vi "总磷测量数据储存.vi"   [LabVIEW 2016, in "斯坦道总磷.lvlib"]
types:
  T1 = cluster{"时间标识":timestamp, "监测值":sgl, "单位":u16, "数据标识":string, "因子编码":u32, "标样参考值":sgl, "F0":sgl, "F1":sgl, "F2":sgl, "F3":sgl, "F4":sgl, "F5":sgl, "F6":sgl, "F7":sgl, "X":sgl, "温度":sgl, "湿度":sgl, "量程标识":string}
  T2 = enum16{"维护数据", "水样测试", "标样核查", "零点核查", "跨度核查", "空白测试", "平行样测试", "加标回收", "空白校准", "标样校准", "初始化（清洗）"}
  T3 = cluster{"运行模式":enum16{"维护模式", "常规模式", "应急模式", "质控模式"}, "质控频次":enum16{"关闭", "每天", "星期一", "星期二", "星期三", "星期四", "星期五", "星期六", "星期日"}, "空白核查时间":u16, "跨度核查时间":u16, "24H周期设置":bool[]}
  T4 = cluster{"系统时间":timestamp, "工作状态":enum16{"空闲", "水样测试", "标样核查", "零点核查", "跨度核查", "空白测试", "平行样测试", "加标回收", "空白校准", "标样校准", "初始化（清洗）"}, "测量模式":enum16{"待机", "连续模式", "周期模式", "定点模式", "受控模式", "手动模式"}, "告警代码":enum16{"无告警", "缺试剂告警", "缺水样告警", "缺蒸馏水告警", "缺标液告警", "仪表漏液告警", "标定异常告警", "超量程告警", "加热异常", "低试剂预警", "超上限告警", "超下限告警", "仪表内部其他异常", "滴定异常告警", "电极异常告警", "量程切换告警", "参数设置告警", "PH电极电位异常", "电导率电极异常", "浊度光度异常", "溶解氧电极异常", "溶解氧光强异常", "温度异常告警", "PH异常告警", "溶解氧异常告警", "电导率异常告警", "浊度异常告警", "叶绿素异常告警", "藻密度异常告警", "蓝绿藻异常告警", "ORP异常告警", "氨氮异常告警", "清洁刷异常告警", "SD卡异常告警", "蓝牙异常告警", "Wifi异常告警", "流程异常告警"}, "故障代码":enum16{"无故障", "电机故障", "温度故障", "通讯故障", "滴定故障"}, "日志代码":u16, "软件版本":u16, "F0":sgl, "F1":sgl, "F2":sgl, "F3":sgl, "T":sgl, "H":sgl, "id":u16, "flowid":u16, "量程":u16, "总磷控温温度1":sgl, "营养盐控温温度2":sgl, "ADC":sgl}
  T5 = enum16{"空闲", "水样测试", "标样核查", "零点核查", "跨度核查", "空白测试", "平行样测试", "加标回收", "空白校准", "标样校准", "初始化（清洗）"}
  T6 = cluster{"因子编码":u32, "单位":u16, "标样参考值":sgl, "水样数据时间":timestamp, "水样实测值":sgl, "水样数据标识":string, "标样数据时间":timestamp, "标样实测值":sgl, "标样数据标识":string, "空白数据时间":timestamp, "空白实测值":sgl, "空白数据标识":string, "零点核查数据时间":timestamp, "零点核查实测值":sgl, "零点核查数据标识":string, "跨度核查数据时间":timestamp, "跨度核查实测值":sgl, "跨度核查数据标识":string, "加标回收数据时间":timestamp, "加标回收实测值":sgl, "加标回收数据标识":string, "平行样数据时间":timestamp, "平行样实测值":sgl, "平行样数据标识":string, "F0":sgl, "F1":sgl, "F2":sgl, "F3":sgl, "F4":sgl, "F5":sgl, "F6":sgl, "F7":sgl, "温度":sgl, "湿度":sgl, "X值":sgl}
  T7 = cluster{"总磷跨度值":dbl, "总磷零点标准液浓度":dbl, "总磷跨度标准液浓度":dbl, "总磷标准液标准浓度":dbl}
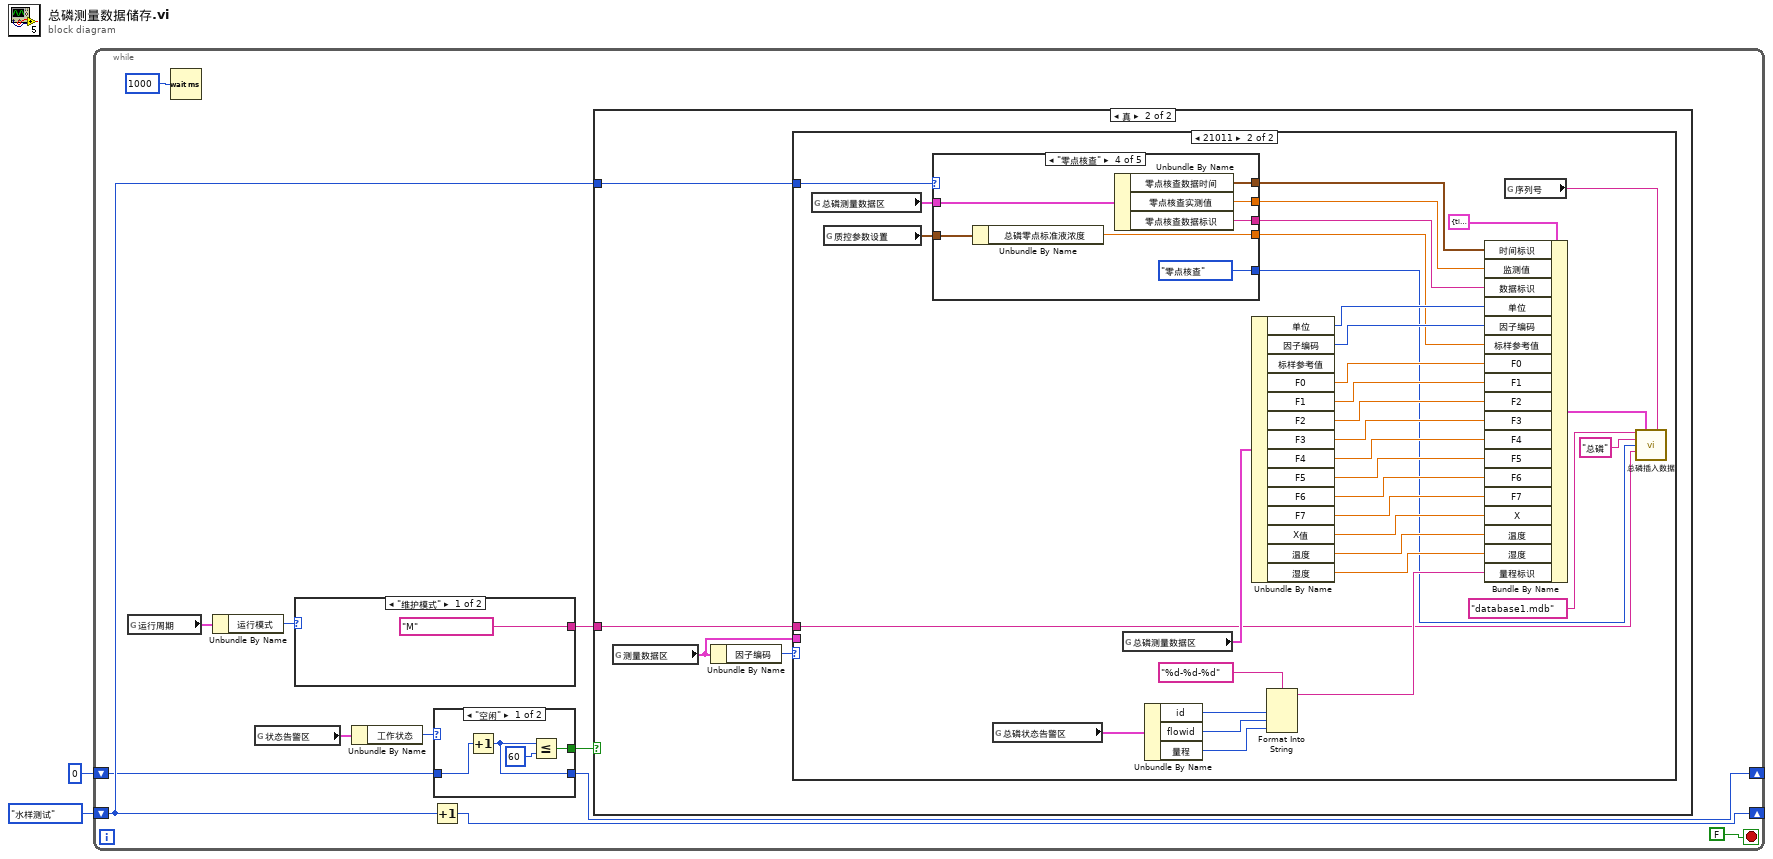
[diagram p0: block diagram]
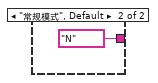
[diagram p3: hidden frame]
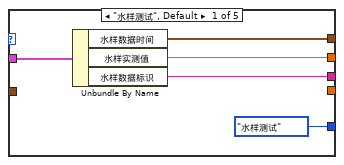
[diagram p6: hidden frame]
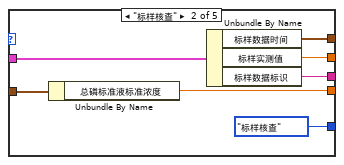
[diagram p7: hidden frame]
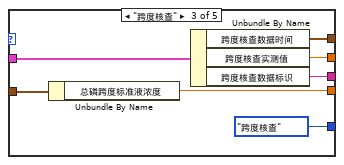
[diagram p8: hidden frame]
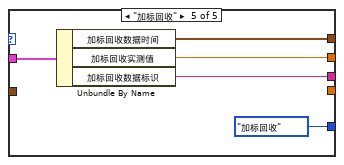
[diagram p9: hidden frame]
diagram:
  n1 = while {
    shift-right: [w12] -> _
    shift-left: enum16{"水样测试", "标样核查", "跨度核查", "零点核查", "加标回收"}."水样测试" ("测量模式") -> [w11]
    shift-right: [w5] -> _
    shift-left: u32 0 ("等待时间（毫秒）") -> [w6]
    stop <- FALSE stop-if-true
    n2 = global read "总磷断电保存全局变量.vi" "运行周期"() -> (w10:T3)
    n3 = Wait (ms)(milliseconds to wait=u32 1000 ("等待时间（毫秒）")) -> ()  [unwired: 1 out]
    n4 = Unbundle By Name(w10) -> ("运行模式"=w9:enum16{"维护模式", "常规模式", "应急模式", "质控模式"})
    n5 = global read "VAR总磷全局变量.vi" "状态告警区"() -> (w8:T4)
    n6 = case shown="\"维护模式\"" w9 {
      tunnel: ["M" ("数据标记表") "N" ("数据标记表")] -> w13
      frame "维护模式" {
      }
      frame "常规模式", Default {
      }
    }
    n7 = Unbundle By Name(w8) -> ("工作状态"=w7:T5)
    n8 = Increment(x=w11) -> (x+1=w12:enum16{"水样测试", "标样核查", "跨度核查", "零点核查", "加标回收"})
    n9 = case shown="\"空闲\"" w7 {
      tunnel: w6 -> [w18 _]
      tunnel: [w17 _] -> w5
      tunnel: [w15 _] -> w4
      frame "空闲" {
        n10 = Increment(x=w18) -> (x+1=w17:u32)
        n11 = Less Or Equal?(x=w17, y=u32 60) -> (x <= y?=w15:bool)
      }
      frame "水样测试", Default {
      }
    }
    n12 = case shown="真" w4 {
      tunnel: w13 -> [_ w22]
      tunnel: w11 -> [_ w21]
      frame False {
      }
      frame True {
        n13 = global read "VAR总磷全局变量.vi" "测量数据区"() -> (w24:T6)
        n14 = Unbundle By Name(w24) -> ("因子编码"=w23:u32)
        n15 = case shown="21011" w23 {
          tunnel: w24 -> [_ _]
          tunnel: w22 -> [_ w29]
          tunnel: w21 -> [_ w28]
          frame Default {
          }
          frame 21011 {
            n16 = global read "VAR总磷全局变量.vi" "总磷测量数据区"() -> (w57:T6)
            n17 = global read "总磷断电保存全局变量.vi" "质控参数设置"() -> (w26:T7)
            n18 = case shown="\"零点核查\"" w28 {
              tunnel: w57 -> [w63 w70 w77 w84 w89]
              tunnel: [w62 w69 w76 w83 w88] -> w33
              tunnel: [w61 w68 w75 w82 w87] -> w34
              tunnel: [w60 w67 w74 w81 w86] -> w35
              tunnel: [T2."水样测试" ("测量模式") T2."标样核查" ("测量模式") T2."跨度核查" ("测量模式") T2."零点核查" ("测量模式") T2."加标回收" ("测量模式")] -> w32
              tunnel: w26 -> [_ w65 w72 w79 _]
              tunnel: [_ w64 w71 w78 _] -> w25
              frame "水样测试", Default {
                n19 = Unbundle By Name(w63) -> ("水样数据时间"=w62:timestamp, "水样实测值"=w61:sgl, "水样数据标识"=w60:string)
              }
              frame "标样核查" {
                n20 = Unbundle By Name(w65) -> ("总磷标准液标准浓度"=w64:dbl)
                n21 = Unbundle By Name(w70) -> ("标样数据时间"=w69:timestamp, "标样实测值"=w68:sgl, "标样数据标识"=w67:string)
              }
              frame "跨度核查" {
                n22 = Unbundle By Name(w72) -> ("总磷跨度标准液浓度"=w71:dbl)
                n23 = Unbundle By Name(w77) -> ("跨度核查数据时间"=w76:timestamp, "跨度核查实测值"=w75:sgl, "跨度核查数据标识"=w74:string)
              }
              frame "零点核查" {
                n24 = Unbundle By Name(w79) -> ("总磷零点标准液浓度"=w78:dbl)
                n25 = Unbundle By Name(w84) -> ("零点核查数据时间"=w83:timestamp, "零点核查实测值"=w82:sgl, "零点核查数据标识"=w81:string)
              }
              frame "加标回收" {
                n26 = Unbundle By Name(w89) -> ("加标回收数据时间"=w88:timestamp, "加标回收实测值"=w87:sgl, "加标回收数据标识"=w86:string)
              }
            }
            n27 = global read "VAR总磷全局变量.vi" "总磷状态告警区"() -> (w27:T4)
            n28 = global read "VAR总磷全局变量.vi" "总磷测量数据区"() -> (w40:T6)
            n29 = Unbundle By Name(w27) -> ("id"=w58:u16, "flowid"=w42:u16, "量程"=w41:u16)
            n30 = Unbundle By Name(w40) -> ("单位"=w56:u16, "因子编码"=w55:u32, "F0"=w54:sgl, "F1"=w53:sgl, "F2"=w52:sgl, "F3"=w51:sgl, "F4"=w50:sgl, "F5"=w49:sgl, "F6"=w48:sgl, "F7"=w47:sgl, "X值"=w46:sgl, "温度"=w45:sgl, "湿度"=w44:sgl)  [unwired: 1 out]
            n31 = Format Into String(format string="%d-%d-%d" ("格式字符串"), w58, w42, w41) -> (resulting string=w43:string)  [unwired: 2 in, 1 out]
            n32 = Bundle By Name(cluster=T1 {"时间标识"=timestamp(0 s since 1904-01-01), "监测值"=0.0, "单位"=0, "数据标识"="", "因子编码"=0, "标样参考值"=0.0, "F0"=0.0, "F1"=0.0, "F2"=0.0, "F3"=0.0, "F4"=0.0, "F5"=0.0, "F6"=0.0, "F7"=0.0, "X"=0.0, "温度"=0.0, "湿度"=0.0, "量程标识"=""} ("data"), "时间标识"=w33, "监测值"=w34, "数据标识"=w35, "单位"=w56, "因子编码"=w55, "标样参考值"=w25, "F0"=w54, "F1"=w53, "F2"=w52, "F3"=w51, "F4"=w50, "F5"=w49, "F6"=w48, "F7"=w47, "X"=w46, "温度"=w45, "湿度"=w44, "量程标识"=w43) -> (w37:T1)
            n33 = global read "VAR总磷全局变量.vi" "序列号"() -> (w36:string)
            n34 = call "总磷插入数据.vi"("database"="database1.mdb", "data"=w37, "SN"=w36, "table"="总磷", "测量模式"=w32, "数据标记表"=w29) -> ()  [unwired: 9 in, 1 out]
          }
        }
      }
    }
  }
